vi "test程序完成后删掉.vi"() -> ()   [LabVIEW 2015]
uses:
  Sub VIs/Digital Image Processing/Digital Image Processing.lvlib
panel:
  in  "Ellipse":T1
  in  "Bounding Rectangle":T2
  out "Image":T3(plugin-control)
  in  "File Path":path
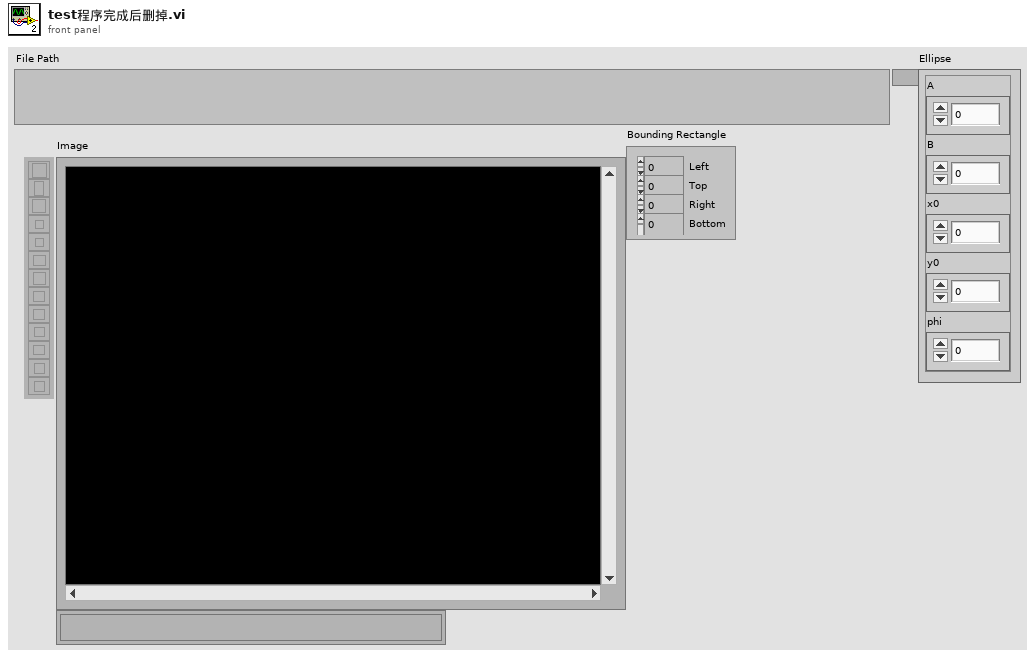
[diagram p1: front panel]
types:
  T1 = cluster{"A":dbl, "B":dbl, "x0":dbl, "y0":dbl, "phi":dbl}
  T2 = cluster{"Left":i32, "Top":i32, "Right":i32, "Bottom":i32}
  T3 = typedef "IMAQ Image.ctl" = refnum<image>
  T4 = typedef "Image Type" = u32
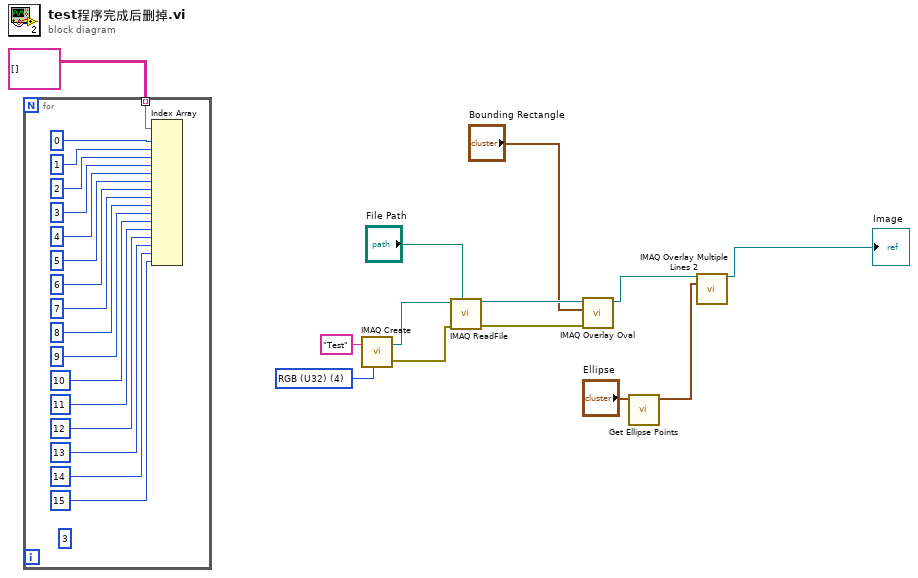
[diagram p0: block diagram]
diagram:
  w1 = T4 4 items=["Grayscale (U8)", "Grayscale (I16)", "Grayscale (SGL)", "Complex (CSG)", "RGB (U32)", "HSL (U32)", "RGB (U64)", "Grayscale (U16)"] ("Image Type")
  n1 = for {
    tunnel: string[][] [] ("数组") -> [w14] mode=indexing
    (unwired) 3 ("索引")
    n2 = Index Array(array=w14, index #1=0 ("索引"), index #2=1 ("索引"), index #3=2 ("索引"), index #4=3 ("索引"), index #5=4 ("索引"), index #6=5 ("索引"), index #7=6 ("索引"), index #8=7 ("索引"), index #9=8 ("索引"), index #10=9 ("索引"), index #11=10 ("索引"), index #12=11 ("索引"), index #13=12 ("索引"), index #14=13 ("索引"), index #15=14 ("索引"), index #16=15 ("索引")) -> ()  [unwired: 16 out]
  }
  n3 = call "IMAQ Create"("Image Name"="Test", "Image Type"=w1) -> ("New Image"=w12:T3, "error out"=w11:errorcluster)  [unwired: 3 in]
  n4 = call "IMAQ ReadFile"("File Path"="File Path", "error in (no error)"=w11, "Image"=w12) -> ("error out"=w6:errorcluster, "Image Out"=w8:T3)  [unwired: 4 in, 3 out]
  n5 = call "IMAQ Overlay Oval"("error in (no error)"=w6, "Bounding Rectangle"="Bounding Rectangle", "Image"=w8) -> ("Image Out"=w5:T3)  [unwired: 7 in, 1 out]
  n6 = call "Get Ellipse Points.vi"("Ellipse"="Ellipse") -> ("Points"=w3:cluster{dbl, dbl}[])  [unwired: 10 in]
  n7 = call "IMAQ Overlay Multiple Lines 2"("Image"=w5, "Line End Points"=w3) -> ("Image Out"=→"Image":T3)  [unwired: 12 in, 1 out]
